vi "gen_stimulus.vi"(7 "Parameters":T1={"Stimulus"={"Type"=enum."Off", "Phase"=0.0, "Amplitude"=[], "Injection point"=enum."Total pose", "Closed loop"=FALSE, "Offset"=[], "Tip -> world"=FALSE, "Frequency"=0.0, "Length"=0.0}, "Goal Filter A"={"Speedup max"=0.0, "Speedup thresh"=0.0, "Speedup nonlin"=0.0, "Filters"=[]}, "Mode controls"={"Hold"=FALSE, "Cancellation"=FALSE, "Goal filter"=FALSE, "Trigger"=FALSE}, "Manipulator type"=enum."Current piezo", "Manipulator calibration"={"Tool offsets"=[[0.0, 0.0, 36200.0]], "Handle light calibration"=[], "Base pivots"=[], "Output pivots"=[], "Length center"=0.0, "Workspace height"=[], "Workspace diameter"=[0.0, 0.0, 36200.0], "Stack travel"=400.0, "Saturation pos"=375.0, "Inverse filters"=[], "Strut length"=0.0}, "Network"={"Remote Host"="", "Send Status"=FALSE, "Send Port"=0, "Recv Commands"=FALSE, "Recv Port"=0}, "Goal Filter B"={"Speedup max"=0.0, "Speedup thresh"=0.0, "Speedup nonlin"=0.0, "Filters"=[]}, "Cancellation"={"KP"={"XY"=0.0, "Rxy"=0.0, "Z"=0.0, "Rz"=0.0}, "KI"=0.0, "KD"={"XY"=0.0, "Rxy"=0.0, "Z"=0.0, "Rz"=0.0}, "Max vel"=20.0, "Max acc"=0.001, "Int error limit"=3.0, "RCM gain"=0.0, "Bypass"=FALSE, "Degraded gain"=0.0}, "Transition time"=0.0, "Estimation"={"Link"={"Measure noise"=[], "Process noise"=[], "Alt process noise"=[], "Alt turnoff cycles"=20, "Innovation limit"=[], "Residue threshold"=0.0, "Enable"=FALSE}, "Handle"={"Measure noise"=[], "Process noise"=[], "State limits"=[], "Innovation limit"=[], "Prediction Lookahead"=0.0, "Enable"=FALSE}}} {"Transition time" format="%_3f"; "Cancellation"."Degraded gain" min=0 max=1 step=0.1 format="%#_3p"; "Cancellation"."RCM gain" min=0 max=1 step=0.1 format="%#_3p"; "Cancellation"."KD"."Rz" min=-1 max=1 step=0.01 format="%#_3p"; "Cancellation"."KD"."Rxy" min=-1 max=1 step=0.01 format="%#_3p"; "Cancellation"."KD"."Z" min=-1 max=1 step=0.01 format="%#_3p"; "Cancellation"."KD"."XY" min=-1 max=1 step=0.01 format="%#_3p"; "Cancellation"."KI" min=0 max=1 step=0.01 format="%#_3p"; "Cancellation"."KP"."Rz" min=-1 max=1 step=0.01 format="%#_3p"; "Cancellation"."KP"."Rxy" min=-1 max=1 step=0.01 format="%#_3p"; "Cancellation"."KP"."Z" min=-1 max=1 step=0.01 format="%#_3p"; "Cancellation"."KP"."XY" min=-1 max=1 step=0.01 format="%#_3p"; "Cancellation"."Max acc" format="%#_3p"; "Goal Filter B"."Filters"."V limit range" format="%_3p"; "Goal Filter B"."Filters"."V limit" format="%_3p"; "Goal Filter B"."Filters"."Upper Q" format="%_3f"; "Goal Filter B"."Filters"."Upper Fc" format="%_3p"; "Goal Filter B"."Filters"."Lower Q" format="%_3f"; "Goal Filter B"."Filters"."Scale factor" format="%_3f"; "Goal Filter B"."Filters"."Lower Fc" format="%_3p"; "Goal Filter B"."Speedup nonlin" format="%_3p"; "Goal Filter B"."Speedup thresh" format="%_3p"; "Goal Filter B"."Speedup max" format="%_3p"; "Manipulator calibration"."Strut length" format="%#_4p"; "Manipulator calibration"."Saturation pos" format="%#.1f"; "Manipulator calibration"."Stack travel" format="%#.1f"; "Manipulator calibration"."Length center" format="%#_4p"; "Manipulator calibration"."Output pivots" format="%#_6f"; "Manipulator calibration"."Base pivots" format="%#_6f"; "Manipulator calibration"."Handle light calibration" format="%#.1f"; "Goal Filter A"."Filters"."V limit range" format="%_3p"; "Goal Filter A"."Filters"."V limit" format="%_3p"; "Goal Filter A"."Filters"."Upper Q" format="%_3f"; "Goal Filter A"."Filters"."Upper Fc" format="%_3p"; "Goal Filter A"."Filters"."Lower Q" format="%_3f"; "Goal Filter A"."Filters"."Scale factor" format="%_3f"; "Goal Filter A"."Filters"."Lower Fc" format="%_3p"; "Goal Filter A"."Speedup nonlin" format="%_3p"; "Goal Filter A"."Speedup thresh" format="%_3p"; "Goal Filter A"."Speedup max" format="%_3p"; "Stimulus"."Length" min=0.0 max=100.0 step=100.0 format="%#_4p"; "Stimulus"."Frequency" min=0.0 step=100.0 format="%#_4g"; "Stimulus"."Offset" format="%#_3p"; "Stimulus"."Amplitude" format="%#_3p"; "Stimulus"."Phase" min=-180.0 max=360.0 step=100.0 format="%#.2f"}, 8 "error in":errorcluster, 9 "Trace index":i32, 10 "Raw handle pose":sgl[][](array[numeric]), 11 "Micron config":T12) -> (0 "error out":errorcluster, 1 "Stimulus":sgl[](array[numeric]), 2 "Stimulus increasing":bool)   [LabVIEW 2014]
uses:
  initialization/micron_config.ctl
  manipulator/squiggle/Host/i2c_interface.ctl
  manipulator/squiggle/Host/fpga_reference.ctl
  Micron params.ctl
  stimulus.ctl
  injection_point.ctl
  filtering/goal_loop_parms.ctl
  mode_conrols.ctl
  manipulator_cal.ctl
  asap/labview/testing/probe_calibration.ctl
  host/network_params.ctl
  cancellation/sq_control_params.ctl
  cancellation/decoupled_gain.ctl
  cancellation/estimation_controls.ctl
  <vilib>/Analysis/baseanly.llb/A x Vector.vi
  <vilib>/Analysis/baseanly.llb/Real A x B.vi
  initialization/micron_globals.vi
  <vilib>/Analysis/Matrix/Numeric/Conversions/Array To Matrix - RA2.vi
  <vilib>/ptbypt/NI_PtbyPt.lvlib
  <vilib>/DAQmx/write.llb/DAQmx Write (Analog 1D DBL NChan 1Samp).vi
  <vilib>/Analysis/Matrix/NI_Matrix.lvlib
  <vilib>/Analysis/NI_AALBase.lvlib
panel:
  in  "DAC min":sgl
  in  "DAC max":sgl=10.0
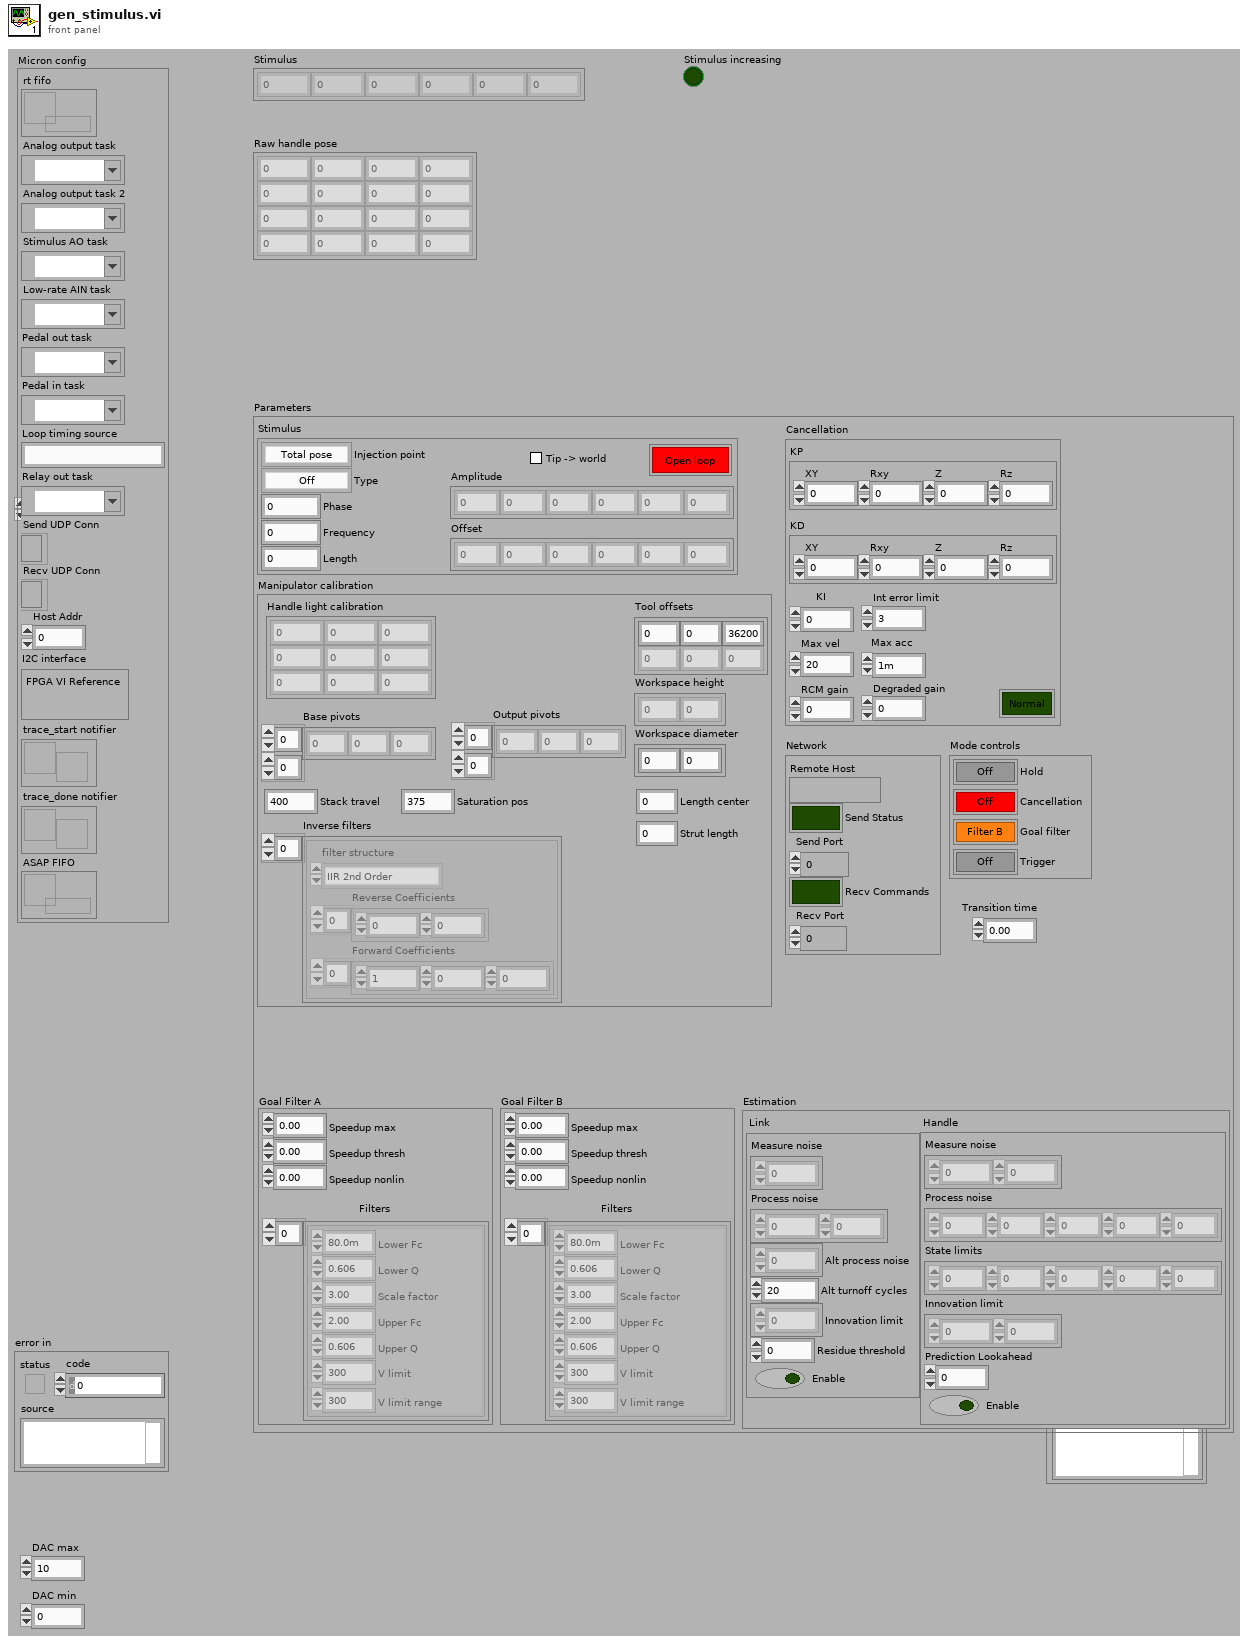
[diagram p1: front panel]
types:
  T1 = typedef "Micron params.ctl" = cluster{"Stimulus":T2, "Goal Filter A":T4, "Mode controls":T5, "Manipulator type":enum16{"Current piezo", "Voltage piezo"}, "Manipulator calibration":T6, "Network":T8, "Goal Filter B":T4, "Cancellation":T9, "Transition time":sgl, "Estimation":T11}
  T2 = typedef "stimulus.ctl" = cluster{"Type":enum16{"Off", "Step", "Sine", "Triangle", "Arbitrary"}, "Phase":dbl, "Amplitude":sgl[], "Injection point":T3, "Closed loop":bool, "Offset":sgl[], "Tip -> world":bool, "Frequency":dbl, "Length":dbl}
  T3 = typedef "injection_point.ctl" = enum16{"Total pose", "V limiter", "Goal ", "Link position", "KF link position", "Inverse kin", "Link goal", "Link error", "Controller", "Output", "Drive", "Light"}
  T4 = typedef "goal_loop_parms.ctl" = cluster{"Speedup max":sgl, "Speedup thresh":sgl, "Speedup nonlin":sgl, "Filters":cluster{"Lower Fc":sgl, "Lower Q":sgl, "Scale factor":sgl, "Upper Fc":sgl, "Upper Q":sgl, "V limit":sgl, "V limit range":sgl}[]}
  T5 = typedef "mode_conrols.ctl" = cluster{"Hold":bool, "Cancellation":bool, "Goal filter":bool, "Trigger":bool}
  T6 = typedef "manipulator_cal.ctl" = cluster{"Tool offsets":sgl[][], "Handle light calibration":T7, "Base pivots":sgl[][], "Output pivots":sgl[][], "Length center":sgl, "Workspace height":sgl[], "Workspace diameter":sgl[], "Stack travel":sgl, "Saturation pos":sgl, "Inverse filters":cluster{"filter structure":enum32{"IIR 2nd Order", "IIR 4th Order"}, "Reverse Coefficients":dbl[], "Forward Coefficients":dbl[]}[], "Strut length":sgl}
  T7 = typedef "probe_calibration.ctl" = sgl[][]
  T8 = typedef "network_params.ctl" = cluster{"Remote Host":string, "Send Status":bool, "Send Port":u16, "Recv Commands":bool, "Recv Port":u16}
  T9 = typedef "sq_control_params.ctl" = cluster{"KP":T10, "KI":sgl, "KD":T10, "Max vel":sgl, "Max acc":sgl, "Int error limit":sgl, "RCM gain":sgl, "Bypass":bool, "Degraded gain":sgl}
  T10 = typedef "decoupled_gain.ctl" = cluster{"XY":sgl, "Rxy":sgl, "Z":sgl, "Rz":sgl}
  T11 = typedef "estimation_controls.ctl" = cluster{"Link":cluster{"Measure noise":dbl[], "Process noise":dbl[], "Alt process noise":dbl[], "Alt turnoff cycles":i32, "Innovation limit":dbl[], "Residue threshold":dbl, "Enable":bool}, "Handle":cluster{"Measure noise":dbl[], "Process noise":dbl[], "State limits":dbl[], "Innovation limit":dbl[], "Prediction Lookahead":sgl, "Enable":bool}}
  T12 = typedef "micron_config.ctl" = cluster{"rt fifo":refnum<k33>, "Analog output task":refnum<k21>, "Analog output task 2":refnum<k21>, "Stimulus AO task":refnum<k21>, "Low-rate AIN task":refnum<k21>, "Pedal out task":refnum<k21>, "Pedal in task":refnum<k21>, "Loop timing source":string, "Relay out task":refnum<k21>, "Send UDP Conn":refnum<k16>, "Recv UDP Conn":refnum<k16>, "Host Addr":u32, "I2C interface":T13, "trace_start notifier":refnum<notifier>, "trace_done notifier":refnum<notifier>, "ASAP FIFO":refnum<k33>}
  T13 = typedef "i2c_interface.ctl" = cluster{"FPGA VI Reference":T14}
  T14 = typedef "fpga_reference.ctl" = refnum<k20>
  T15 = enum16{"Off", "Step", "Sine", "Triangle", "Arbitrary"}
  T16 = typedef "NI_Matrix.lvlib/RealMatrix.ctl" = dbl[][]
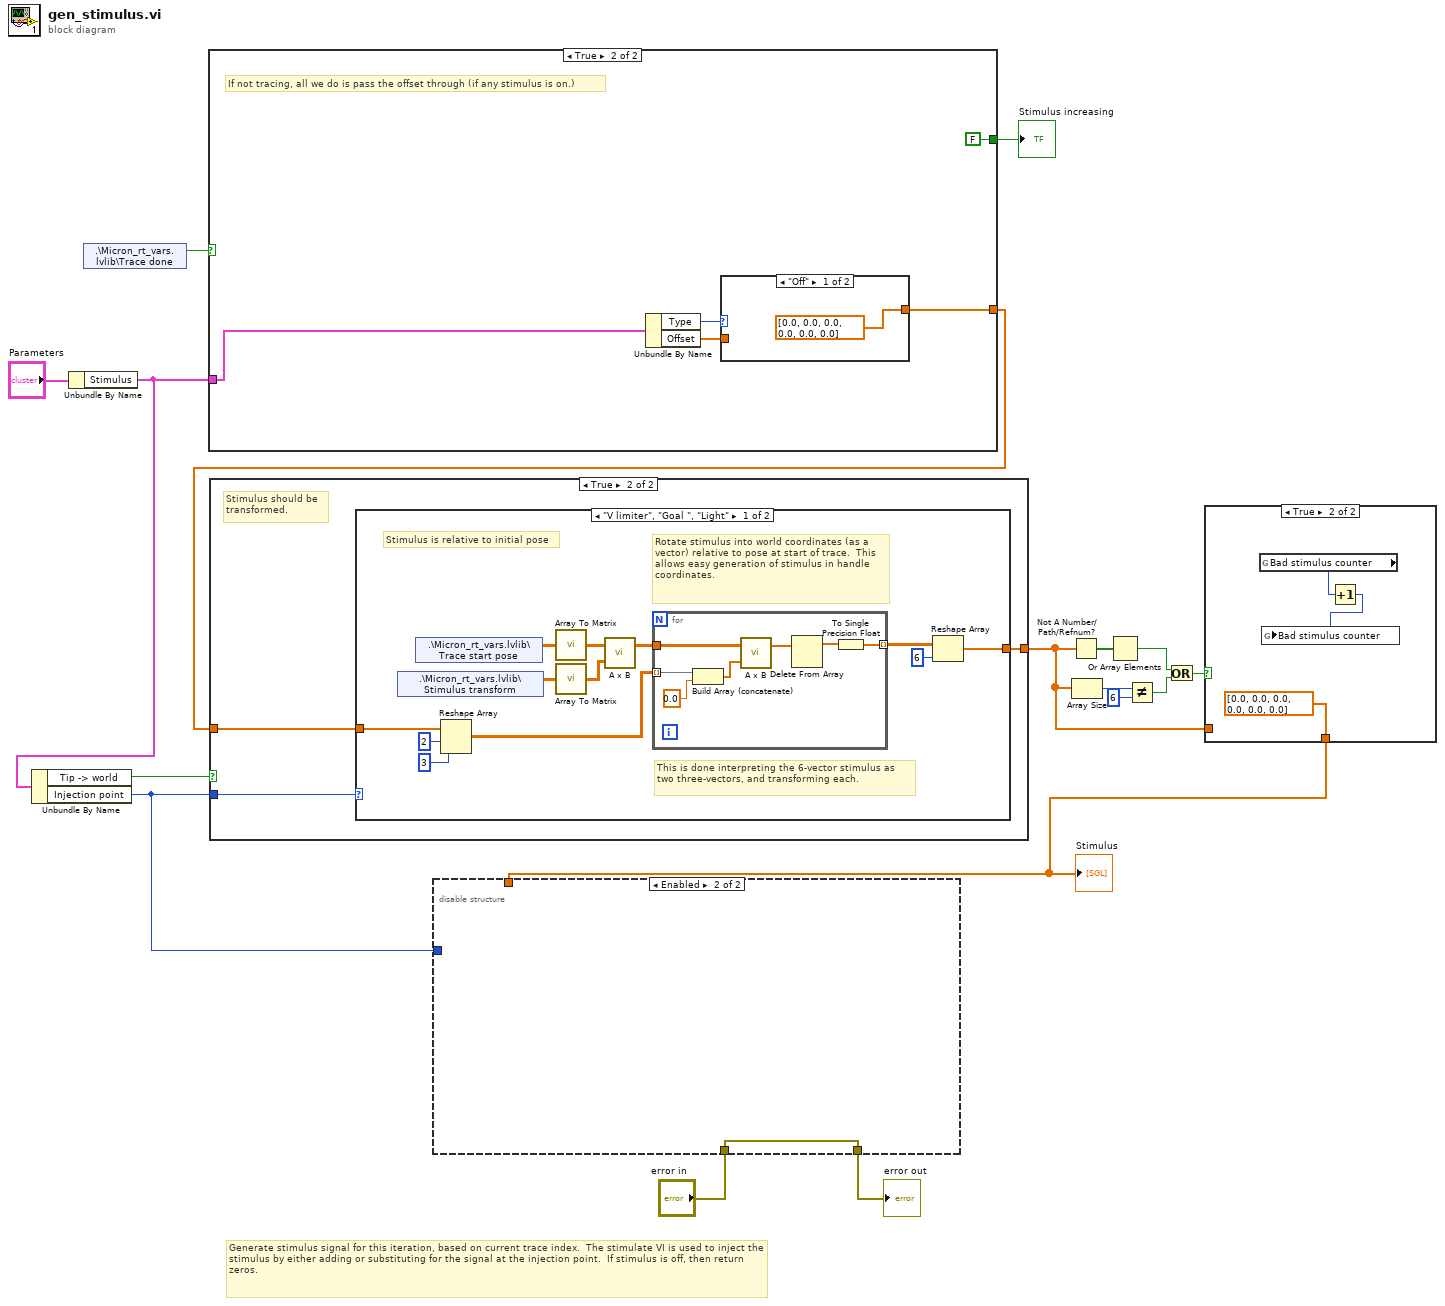
[diagram p0: block diagram]
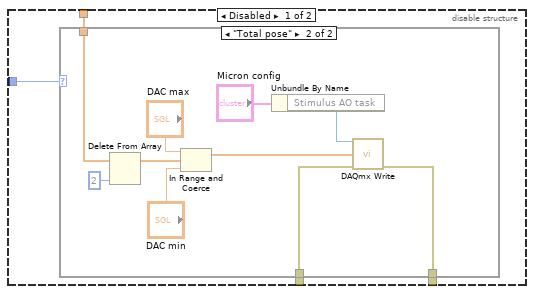
[diagram p3: hidden frame]
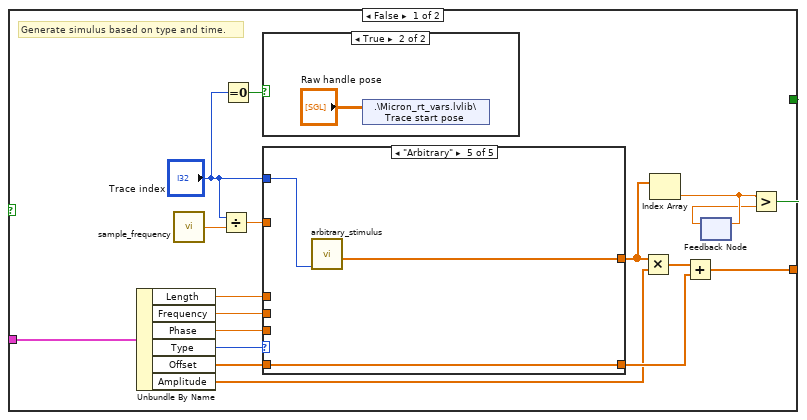
[diagram p7: hidden frame]
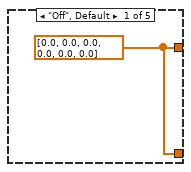
[diagram p9: hidden frame]
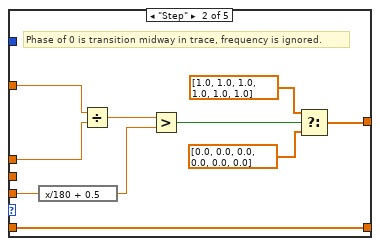
[diagram p10: hidden frame]
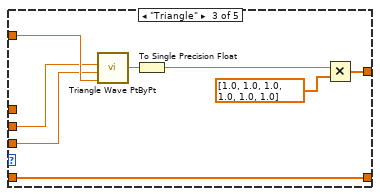
[diagram p11: hidden frame]
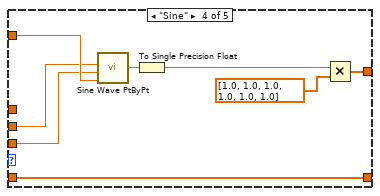
[diagram p12: hidden frame]
diagram:
  # "Generate stimulus signal for this iteration, based on current trace index.  The stimulate VI is used to inject the stimulus by either adding or substituting for the signal at the injection point.  If stimulus is off, then return zeros."
  n1 = Unbundle By Name("Parameters") -> ("Stimulus"=w12:T2)
  n2 = Unbundle By Name(w12) -> ("Tip -> world"=w14:bool, "Injection point"=w13:T3)
  n3 = shared-variable ".\\Micron_rt_vars.lvlib\\Trace done"() -> (w17:bool)  [unwired: 2 out]
  n4 = case shown="True" w17 {
    tunnel: [w32 w69] -> w2
    tunnel: w12 -> [w28 w68]
    tunnel: [w20 FALSE] -> w10
    frame False {
      # "Generate simulus based on type and time."
      n5 = Unbundle By Name(w28) -> ("Length"=w24:dbl, "Frequency"=w25:dbl, "Phase"=w26:dbl, "Type"=w34:T15, "Offset"=w31:sgl[], "Amplitude"=w29:sgl[])
      n6 = call "sample_frequency.vi"() -> ("Sample frequency"=w27:dbl)
      n7 = Divide(x="Trace index", y=w27) -> (x/y=w35:dbl)
      n8 = Equal To 0?(x="Trace index") -> (x = 0?=w19:bool)
      n9 = case shown="True" w19 {
        frame False {
        }
        frame True {
          n10 = shared-variable ".\\Micron_rt_vars.lvlib\\Trace start pose"("Raw handle pose") -> ()  [unwired: 2 out]
        }
      }
      n11 = case shown="\"Arbitrary\"" w34 {
        tunnel: w35 -> [_ w41 w55 w63 _]
        tunnel: [w37 w45 w51 w59 w66] -> w23
        tunnel: w31 -> [_ w43 w50 w58 w65]
        tunnel: [w37 w43 w50 w58 w65] -> w30
        tunnel: w26 -> [_ w42 w49 w57 _]
        tunnel: w25 -> [_ _ w48 w56 _]
        tunnel: w24 -> [_ w40 _ _ _]
        tunnel: "Trace index" -> [_ _ _ _ w64]
        frame "Off", Default {
          w37 = sgl[] [0.0, 0.0, 0.0, 0.0, 0.0, 0.0] ("Amplitude")
        }
        frame "Step" {
          # "Phase of 0 is transition midway in trace, frequency is ignored."
          n12 = expression code="x/180 + 0.5"(w42) -> (w38:dbl)
          n13 = Divide(x=w41, y=w40) -> (x/y=w39:dbl)
          n14 = Greater?(x=w39, y=w38) -> (0:w47:bool)
          n15 = Select(t=sgl[] [1.0, 1.0, 1.0, 1.0, 1.0, 1.0] ("Amplitude"), s=w47, f=sgl[] [0.0, 0.0, 0.0, 0.0, 0.0, 0.0] ("Amplitude")) -> (s? t:f=w45:sgl[])
        }
        frame "Triangle" {
          n16 = call <vilib>:"Triangle Wave PtByPt.vi"("time"=w55, "phase"=w49, "frequency"=w48) -> ("triangle wave"=w54:dbl)  [unwired: 1 in]
          n17 = To Single Precision Float(number=w54) -> (single precision float=w53:sgl)
          n18 = Multiply(x=w53, y=sgl[] [1.0, 1.0, 1.0, 1.0, 1.0, 1.0] ("Amplitude")) -> (x*y=w51:sgl[])
        }
        frame "Sine" {
          n19 = call <vilib>:"Sine Wave PtByPt.vi"("time"=w63, "phase"=w57, "frequency"=w56) -> ("sine wave"=w62:dbl)  [unwired: 1 in]
          n20 = To Single Precision Float(number=w62) -> (single precision float=w61:sgl)
          n21 = Multiply(x=w61, y=sgl[] [1.0, 1.0, 1.0, 1.0, 1.0, 1.0] ("Amplitude")) -> (x*y=w59:sgl[])
        }
        frame "Arbitrary" {
          n22 = call "arbitrary_stimulus.vi"("index"=w64) -> ("Value"=w66:sgl[])  [unwired: 2 in, 8 out]
        }
      }
      n23 = Multiply(x=w23, y=w29) -> (x*y=w33:sgl[])
      n24 = Index Array(array=w23) -> (element=w22:sgl)  [unwired: 1 in]
      n25 = Add(x=w33, y=w30) -> (x+y=w32:sgl[])
      n26 = feedback-in #1(w22) -> ()
      n27 = feedback #1() -> (w21:sgl)  [unwired: 1 in]
      n28 = Greater?(x=w22, y=w21) -> (0:w20:bool)
    }
    frame True {
      # "If not tracing, all we do is pass the offset through (if any stimulus is on.)"
      n29 = Unbundle By Name(w68) -> ("Type"=w71:T15, "Offset"=w70:sgl[])
      n30 = case shown="\"Off\"" w71 {
        tunnel: [sgl[] [0.0, 0.0, 0.0, 0.0, 0.0, 0.0] ("Amplitude") w73] -> w69
        tunnel: w70 -> [_ w73]
        frame "Off" {
        }
        frame Default {
        }
      }
    }
  }
  "Stimulus increasing" <- w10
  n31 = case shown="True" w14 {
    tunnel: w2 -> [w74 w76]
    tunnel: [w74 w77] -> w4
    tunnel: w13 -> [_ w75]
    frame False {
      # "No coordinate transformation on stimulus."
    }
    frame True {
      # "Stimulus should be\ntransformed."
      n32 = case shown="\"V limiter\", \"Goal \", \"Light\"" w75 {
        tunnel: [w83 w97] -> w77
        tunnel: w76 -> [w89 w97]
        frame "V limiter", "Goal ", "Light" {
          # "This is done interpreting the 6-vector stimulus as two three-vectors, and transforming each."
          # "Rotate stimulus into world coordinates (as a vector) relative to pose at start of trace.  This allows easy generation of stimulus in handle coordinates."
          # "Stimulus is relative to initial pose"
          n33 = shared-variable ".\\Micron_rt_vars.lvlib\\Stimulus transform"() -> (w81:sgl[][])  [unwired: 2 out]
          n34 = shared-variable ".\\Micron_rt_vars.lvlib\\Trace start pose"() -> (w82:sgl[][])  [unwired: 2 out]
          n35 = Reshape Array(w89, 2 ("dimension size"), 3 ("dimension size")) -> (w86:sgl[][])
          n36 = call-poly <vilib>:"Array To Matrix.vi"("Real 2D Array"=w82) -> ("Real Matrix"=w80:T16)
          n37 = call-poly <vilib>:"Array To Matrix.vi"("Real 2D Array"=w81) -> ("Real Matrix"=w79:T16)
          n38 = call-poly <vilib>:"A x B.vi"("B"=w79, "A"=w80) -> ("A x B"=w78:T16)  [unwired: 1 out]
          n39 = for {
            tunnel: [w92] -> w85 mode=indexing
            tunnel: w78 -> [w91]
            tunnel: w86 -> [w90] mode=indexing
            n40 = Build Array (concatenate)(w90, sgl 0.0 ("Numeric")) -> (w96:sgl[])
            n41 = call-poly <vilib>:"A x B.vi"("Vector"=w96, "A"=w91) -> ("A x Vector"=w94:dbl[])  [unwired: 1 out]
            n42 = Delete From Array(array=w94) -> (array with subset deleted=w93:dbl[])  [unwired: 2 in, 1 out]
            n43 = To Single Precision Float(number=w93) -> (single precision float=w92:sgl[])
          }
          n44 = Reshape Array(w85, 6 ("dimension size")) -> (w83:sgl[])
        }
        frame Default {
          # "In 3DOF, we used to run the stimulus through the inverse kinematics, but that was easier with the linear\napproximate kinematics.  For now, don't transform link-length stimulus at all.  Perhaps the goal loop\nshould compute an approximate linearization.\n\nFor \"Total pose\" injection, the transform is done by stimulate_pose.vi"
        }
      }
    }
  }
  n45 = Not A Number/Path/Refnum?(number/path/refnum=w4) -> (NaN/Path/Refnum?=w7:bool[])
  n46 = Array Size(array=w4) -> (size(s)=w9:i32)
  n47 = Or Array Elements(Boolean array=w7) -> (logical OR=w5:bool)
  n48 = Not Equal?(x=w9, y=6) -> (x != y?=w6:bool)
  n49 = Or(x=w5, y=w6) -> (x .or. y?=w1:bool)
  n50 = case shown="True" w1 {
    tunnel: w4 -> [w98 _]
    tunnel: [w98 sgl[] [0.0, 0.0, 0.0, 0.0, 0.0, 0.0] ("Amplitude")] -> w3
    frame False {
    }
    frame True {
      n51 = global read "micron_globals.vi" "Bad stimulus counter"() -> (w100:i32)
      n52 = Increment(x=w100) -> (x+1=w99:i32)
      n53 = global write "micron_globals.vi" "Bad stimulus counter"(w99) -> ()
    }
  }
  "Stimulus" <- w3
  n54 = disable-structure shown="Enabled" {
    disable-tunnel: "error in" -> [w105 w117]
    disable-tunnel: [w104 w117] -> w15
    disable-tunnel: w3 -> [w103 _]
    disable-tunnel: w13 -> [w102 _]
    frame Disabled {
      n55 = case shown="\"DAC\"" w102 {
        tunnel: w103 -> [_ w112]
        tunnel: w105 -> [w106 w114]
        tunnel: [w106 w113] -> w104
        frame "Total pose", Default {
        }
        frame "Total pose" {
          n56 = Delete From Array(array=w112, index=2) -> (array with subset deleted=w110:sgl[])  [unwired: 1 in, 1 out]
          n57 = In Range and Coerce(upper limit="DAC max", x=w110, lower limit="DAC min") -> (coerced(x)=w107:sgl[])  [unwired: 1 out]
          n58 = Unbundle By Name("Micron config") -> ("Stimulus AO task"=w116:refnum<k21>)
          n59 = call-poly <vilib>:"DAQmx Write.vi"("task/channels in"=w116, "data"=w107, "error in"=w114) -> ("error out"=w113:errorcluster)  [unwired: 1 in, 11 out]
        }
      }
    }
    frame Enabled {
    }
  }
  "error out" <- w15
